vi "SaveCompiled.vi"() -> ()   [LabVIEW 2011]
panel:
  out "File String":string
  in  "Chapter":string="Chapter(DopplerCooling,\n10100000 00000000 00000000)\nChapter(Pump,\n01000000 00000000 00000000)\nChapter(Pulsed,\n00100000 00000000 00000000,\n00000100 00000000 00000000,\n00000000 10000000 00000000,\n01000000 00000000 01000000)\nChapter(Zero,\n00000000 00000000 00000000)\nChapter(One,\n11111111 11111111 11111111)\n"
  in  "Sequence":string="Zero(1)\nOne(1)\nZero(1)\nOne(1)\nZero(1)\nOne(1)\nZero(1)\nOne(1)\nZero(1)\nOne(1)\n"
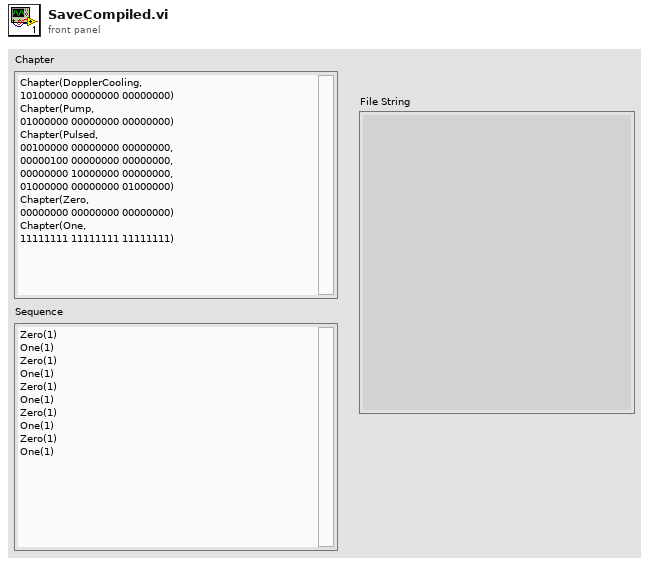
[diagram p1: front panel]
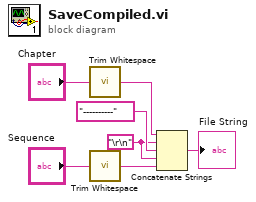
[diagram p0: block diagram]
diagram:
  w1 = "\r\n"
  n1 = call <vilib>:"Trim Whitespace.vi"("string"="Chapter") -> ("trimmed string"=w4:string)  [unwired: 1 in]
  n2 = call <vilib>:"Trim Whitespace.vi"("string"="Sequence") -> ("trimmed string"=w2:string)  [unwired: 1 in]
  n3 = Concatenate Strings(w4, w1, "----------" ("string"), w1, w2) -> (→"File String":string)
